vi "convertGyroRawData.vi"(0 "raw x":i16, 7 "raw y":i16, 11 "raw z":i16) -> (4 "x":sgl, 8 "y":sgl, 15 "z":sgl)   [LabVIEW 2023]
panel:
  in  "scale [dps]":sgl=250.0 format="%#_13g"
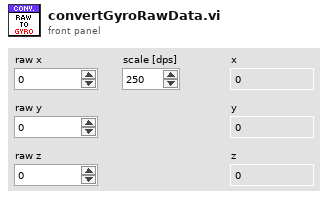
[diagram p1: front panel]
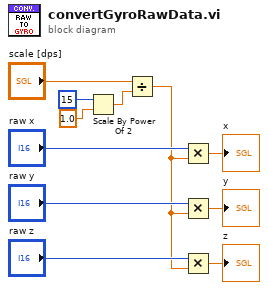
[diagram p0: block diagram]
diagram:
  n1 = Scale By Power Of 2(n=i16 15, x=sgl 1.0) -> (x*2^n=w8:sgl)
  n2 = Divide(x="scale [dps]", y=w8) -> (x/y=w1:sgl)
  n3 = Multiply(x="raw x", y=w1) -> (x*y=→"x":sgl)
  n4 = Multiply(x="raw y", y=w1) -> (x*y=→"y":sgl)
  n5 = Multiply(x="raw z", y=w1) -> (x*y=→"z":sgl)
